vi "Set Test Group.vi"(0 "Test Group Manager in":refnum<class "Test Group Manager.lvclass">, 2 "Test Group Name":string, 3 "DPD LUT Name":string, 4 "Input Power":string, 5 "error in (no error)":errorcluster) -> (14 "Test Group Manager out":refnum<class "Test Group Manager.lvclass">, 19 "error out":errorcluster)   [LabVIEW 2016, in "Test Group Manager.lvlib" / "Test Group Manager.lvclass"]
uses:
  Test Group Manager.lvclass
  Test Group Manager.lvclass/Test Group Manager.ctl
  Includes/Test Group/Test Group.lvclass
  Protected Methods/Read Test Group Database.vi
  Protected Methods/Write Test Group Database.vi
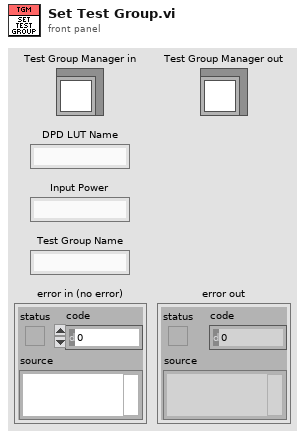
[diagram p1: front panel]
types:
  T1 = cluster{"DPD LUT Name":string, "Input Power":string}
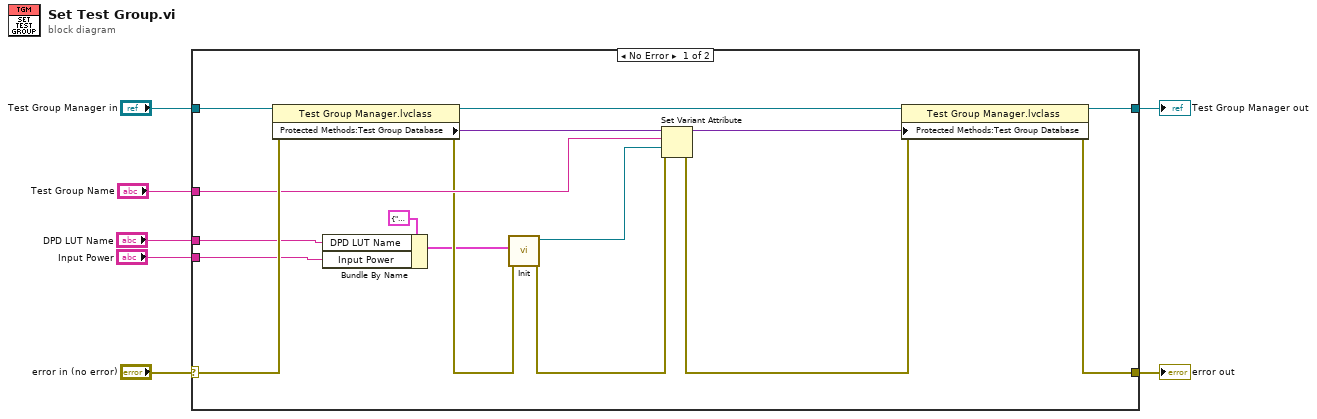
[diagram p0: block diagram]
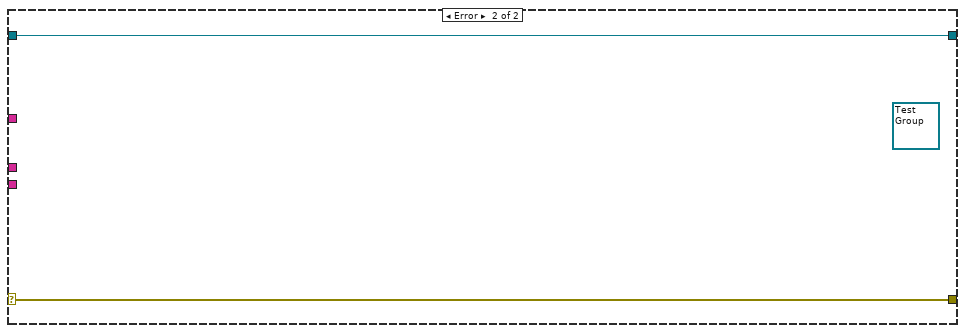
[diagram p2: hidden frame]
diagram:
  n1 = case shown="No Error" "error in (no error)" {
    selector: "error in (no error)" -> [w23 w25]
    tunnel: [w12 w25] -> w6
    tunnel: [w10 w24] -> w4
    tunnel: "Test Group Manager in" -> [w22 w24]
    tunnel: "Test Group Name" -> [w20 _]
    tunnel: "DPD LUT Name" -> [w16 _]
    tunnel: "Input Power" -> [w15 _]
    frame No Error {
      n2 = property class="Test Group Manager.lvclass"(reference=w22, error in=w23) -> (reference out=w11:refnum<class "Test Group Manager.lvclass">, error out=w19:errorcluster, "Protected Methods:Test Group Database"=w21:variant)
      n3 = Bundle By Name(cluster=T1 {"DPD LUT Name"="", "Input Power"=""} ("Test Group Data"), "DPD LUT Name"=w16, "Input Power"=w15) -> (w17:T1)
      n4 = call "Init.vi"("error in (no error)"=w19, "Test Group Data"=w17) -> ("error out"=w14:errorcluster, "data value reference"=w8:refnum<data-value>)  [unwired: 8 in]
      n5 = Set Variant Attribute(Variant=w21, name=w20, value=w8, error in=w14) -> (Variant out=w9:variant, error out=w13:errorcluster)  [unwired: 1 out]
      n6 = property class="Test Group Manager.lvclass"(reference=w11, error in=w13, "Protected Methods:Test Group Database"=w9) -> (reference out=w10:refnum<class "Test Group Manager.lvclass">, error out=w12:errorcluster)
    }
    frame Error {
      (unwired) refnum<class "Test Group.lvclass"> refnum ("Test Group Manager.lvlib:Test Group.lvclass")
    }
  }
  "error out" <- w6
  "Test Group Manager out" <- w4
